vi "Read CS.vi"(8 "error in (no error)":errorcluster, 11 "Device Configuration in":refnum<class "Device Configuration.lvclass">) -> (0 "error out":errorcluster, 2 "CS":string(combo), 3 "Device Configuration out":refnum<class "Device Configuration.lvclass">)   [LabVIEW 2014, in "Device Configuration.lvclass"]
uses:
  Device Configuration.lvclass
  <vilib>/NI/Configuration Framework/serializable configuration/NISE_CEF_serializable configuration.lvclass
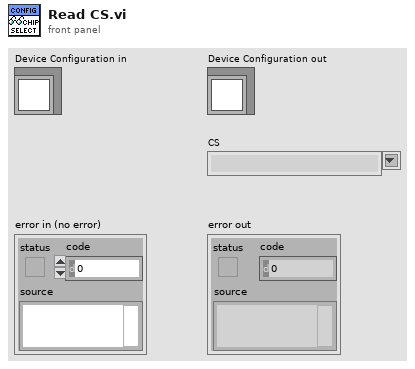
[diagram p1: front panel]
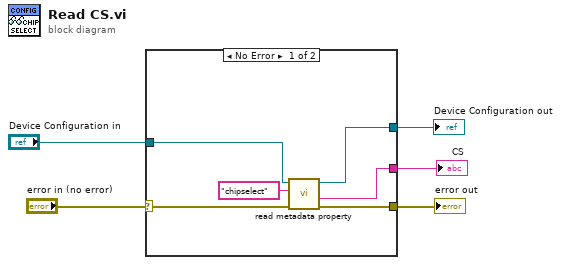
[diagram p0: block diagram]
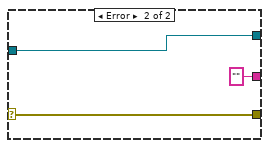
[diagram p2: hidden frame]
diagram:
  n1 = case shown="No Error" "error in (no error)" {
    selector: "error in (no error)" -> [w10 w14]
    tunnel: "Device Configuration in" -> [w9 w13]
    tunnel: [w8 w14] -> w3
    tunnel: [w7 "" ("value")] -> w2
    tunnel: [w6 w13] -> w1
    frame No Error {
      n2 = call <vilib>:"read metadata property.vi"("error in"=w10, "key"="chipselect", "configuration in"=w9) -> ("error out"=w8:errorcluster, "value"=w7:string, "configuration out"=w6:refnum<class "Device Configuration.lvclass">)  [unwired: 5 in, 1 out]
    }
    frame Error {
    }
  }
  "error out" <- w3
  "Device Configuration out" <- w1
  "CS" <- w2
